vi "Force Base Class.vi"(8 "error in (no error)":errorcluster, 11 "Carya Config in":refnum<class "Carya Config.lvclass">) -> (0 "error out":errorcluster, 2 "Carya Config out":refnum<class "Carya Config.lvclass">, 3 "Carya Config out":refnum<class "Carya Config.lvclass">)   [LabVIEW 2013, in "Carya Config.lvclass"]
doc: "Copyright 2018, Carya Automatisering, Wiebe Walstra."
uses:
  Carya Config.lvclass
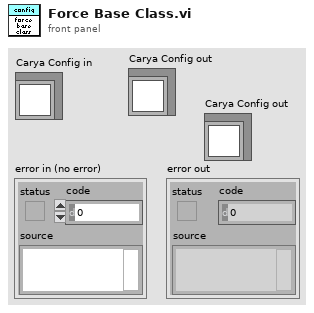
[diagram p1: front panel]
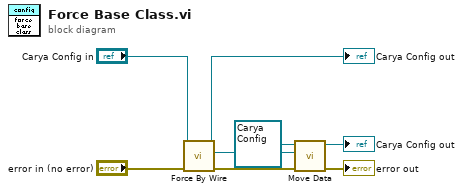
[diagram p0: block diagram]
diagram:
  n1 = call-dynamic "Force By Wire.vi"("error in (no error)"="error in (no error)", "Carya Config in"="Carya Config in") -> ("error out"=w4:errorcluster, 2:"Carya Config out"=w5:refnum<class "Carya Config.lvclass">, 3:"Carya Config out"=→"Carya Config out":refnum<class "Carya Config.lvclass">)  [unwired: 7 in]
  n2 = call "Move Data.vi"("error in (no error)"=w4, "Carya Config source"=w5, "Carya Config dest"=refnum<class "Carya Config.lvclass"> refnum ("Carya Config.lvclass")) -> ("error out"=→"error out":errorcluster, "Carya Config out"=→"Carya Config out":refnum<class "Carya Config.lvclass">)  [unwired: 7 in]
